vi "fftw__execute_poly.vi"   [LabVIEW 2020, in "FFTWDLL.lvlib"]
doc: "Execute FFTW plan."
uses:
  FFTWDLL.lvlib
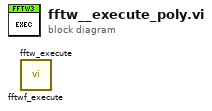
[diagram p0: block diagram]
diagram:
  n1 = call "fftwf_execute.vi"() -> ()  [unwired: 10 in, 2 out]
  n2 = call "fftw_execute.vi"() -> ()  [unwired: 10 in, 2 out]
